vi "cmc_array_to_cluster.vi"() -> ()   [LabVIEW 2011]
panel:
  in  "Delay Time (s)":dbl=1.0
  in  "STOP":bool
  out "Array":dbl[][](array[numeric]) format="%#_4g"
  out "Cluster 2":T1 {"Average of Row 4" scale=0.0..1.0; "Gauge 4" scale=0.0..1.0; "Gauge 3" scale=0.0..1.0; "Gauge 2" scale=0.0..1.0; "Gauge" scale=0.0..1.0}
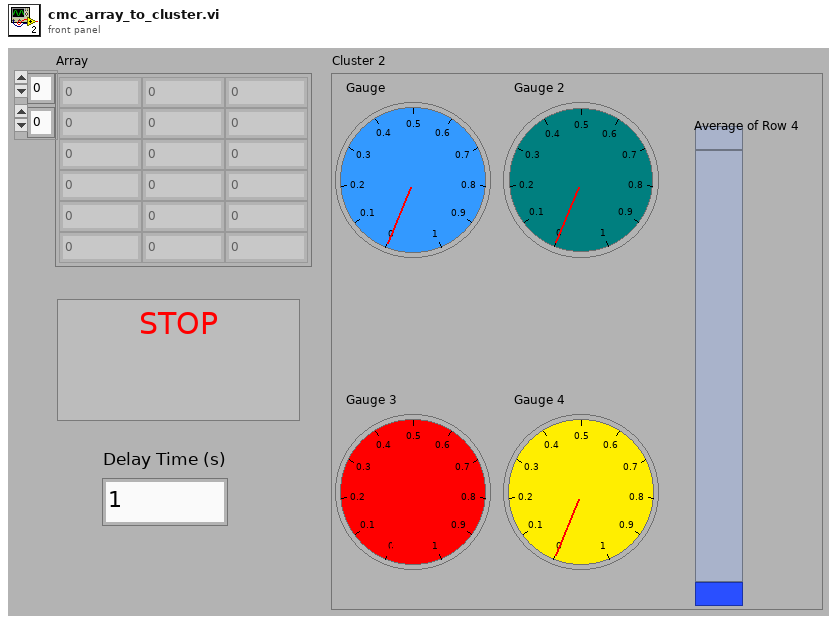
[diagram p1: front panel]
types:
  T1 = cluster{"Gauge":dbl, "Gauge 2":dbl, "Gauge 3":dbl, "Average of Row 4":dbl, "Gauge 4":dbl}
  T2 = cluster{"[0]":dbl, "[1]":dbl, "[2]":dbl, "[3]":dbl, "[4]":dbl}
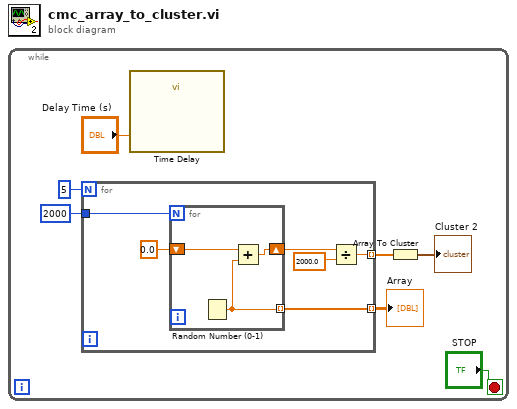
[diagram p0: block diagram]
diagram:
  n1 = while {
    stop <- "STOP" stop-if-true
    n2 = for {
      N: 5 -> [_]
      tunnel: 2000 -> [w13]
      tunnel: [w10] -> w3 mode=indexing
      tunnel: [w8] -> w4 mode=indexing
      n3 = for {
        N: w13 -> [_]
        shift-right: [w14] -> w9
        shift-left: 0.0 ("number: 0 to 1") -> [w15]
        tunnel: [w16] -> w10 mode=indexing
        n4 = Random Number (0-1)() -> (number: 0 to 1=w16:dbl)
        n5 = Add(x=w15, y=w16) -> (x+y=w14:dbl)
      }
      n6 = Divide(x=w9, y=2000.0) -> (x/y=w8:dbl)
    }
    "Array" <- w3
    n7 = call "Time Delay"("Delay Time (s)"="Delay Time (s)") -> ()  [unwired: 10 in, 1 out]
    n8 = Array To Cluster(array=w4) -> (cluster=→"Cluster 2":T2)
  }
